vi "TAT_Com_PLC.vi"() -> ()   [LabVIEW 2017]
uses:
  <vilib>/NI/Modbus Library/API/Wrapper/Create TCP Master.vi
  <vilib>/NI/Modbus Library/API/Master/Modbus Master.lvclass
  <vilib>/NI/Modbus Library/API/Wrapper/API Main.lvlib
panel:
  out "Array":i32[](array[numeric])
  out "PLC STATUS":bool
  in  "error in":errorcluster
  in  "stop":bool
  # "Ass & Leak"
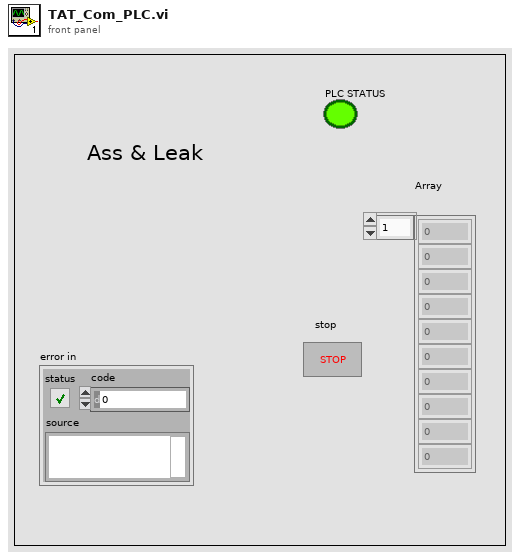
[diagram p1: front panel]
types:
  T1 = enum32{"invalid app kind", "Development System", "Run Time System", "Student Edition", "Embedded LabVIEW", "Evaluation", "Custom"}
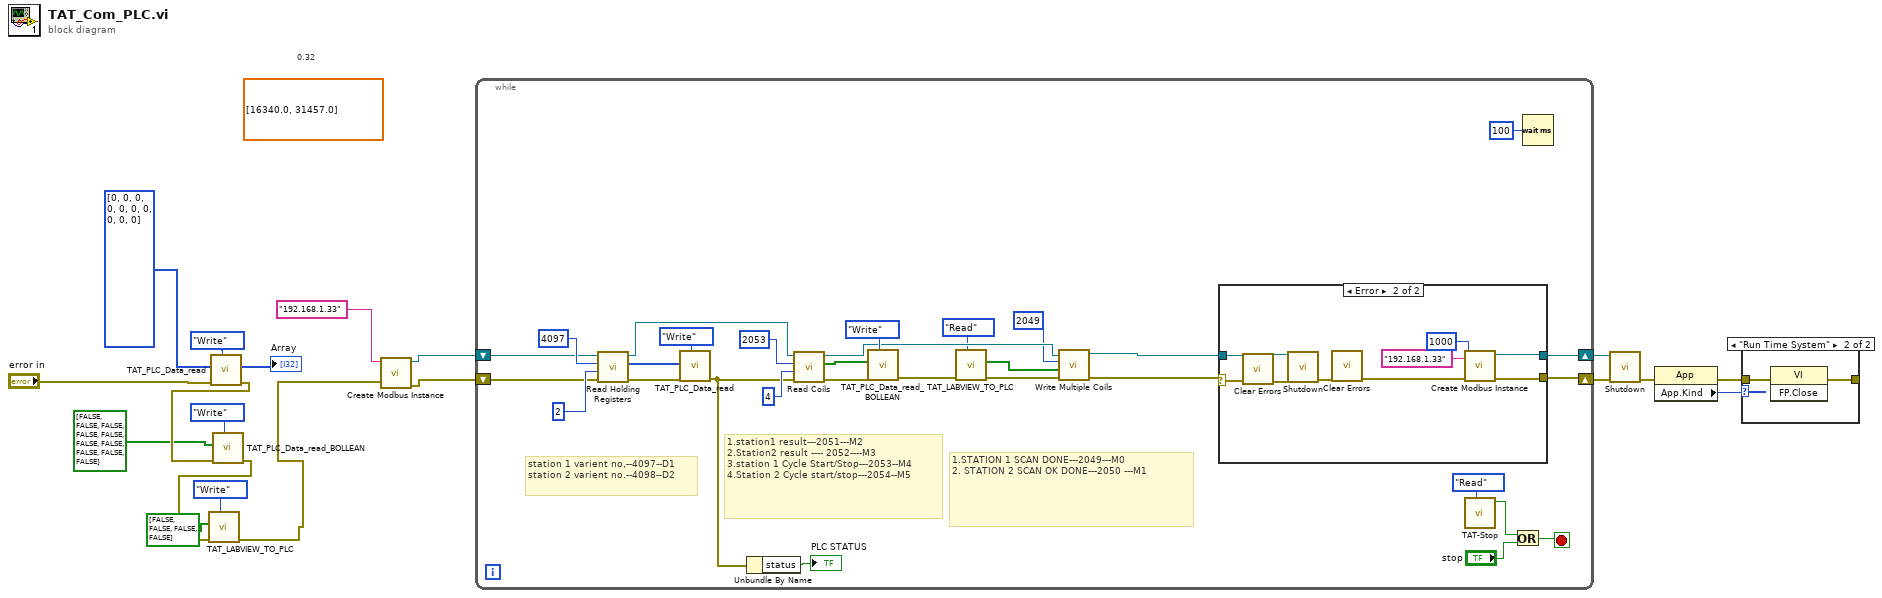
[diagram p0: block diagram]
diagram:
  (unwired) dbl[] [16340.0, 31457.0] ("register values")
  # "0.32"
  n1 = call "TAT_PLC_Data_read.vi"("Enum"=enum16{"Read", "Write"}."Write", "error in (no error)"="error in", "Array"=i64[] [0, 0, 0, 0, 0, 0, 0, 0, 0, 0] ("Array 3")) -> ("error out"=w6:errorcluster, "Array 2"=→"Array":u16[])  [unwired: 7 in]
  n2 = call "TAT_PLC_Data_read_BOLLEAN.vi"("Enum"=enum16{"Read", "Write"}."Write", "error in (no error)"=w6, "Array"=bool[] [FALSE, FALSE, FALSE, FALSE, FALSE, FALSE, FALSE, FALSE, FALSE, FALSE]) -> ("error out"=w2:errorcluster)  [unwired: 7 in, 1 out]
  n3 = call "TAT_LABVIEW_TO_PLC.vi"("Enum"=enum16{"Read", "Write"}."Write", "error in (no error)"=w2, "Array"=bool[] [FALSE, FALSE, FALSE, FALSE]) -> ("error out"=w3:errorcluster)  [unwired: 7 in, 1 out]
  n4 = call-poly <vilib>:"Create Modbus Instance.vi"("error in"=w3, "address"="192.168.1.33") -> ("error out"=w13:errorcluster, "TCP master instance"=w12:refnum<class "Modbus Master.lvclass">)  [unwired: 8 in]
  n5 = while {
    shift-right: [w47] -> w18
    shift-left: w12 -> [w42]
    shift-right: [w46] -> w17
    shift-left: w13 -> [w43]
    stop <- w48 stop-if-true
    # "1.STATION 1 SCAN DONE---2049---M0\n2. STATION 2 SCAN OK DONE---2050 ---M1"
    # "1.station1 result---2051---M2\n2.Station2 result ---- 2052----M3\n3.station 1 Cycle Start/Stop---2053--M4\n4.Station 2 Cycle start/stop---2054--M5"
    # "station 1 varient no,--4097--D1\nstation 2 varient no.--4098--D2"
    n6 = call-dynamic "Read Holding Registers.vi"("error in"=w43, "number of inputs"=u16 2, "starting address"=u16 4097, "Modbus master in"=w42) -> ("error out"=w37:errorcluster, "register values"=w39:u16[], "Modbus master out"=w33:refnum<class "Modbus Master.lvclass">)  [unwired: 5 in]
    n7 = call "TAT_PLC_Data_read.vi"("Enum"=enum16{"Read", "Write"}."Write", "error in (no error)"=w37, "Array"=w39) -> ("error out"=w34:errorcluster)  [unwired: 7 in, 1 out]
    n8 = Unbundle By Name(w34) -> ("status"=→"PLC STATUS":bool)
    n9 = call-dynamic "Read Coils.vi"("error in"=w34, "number of inputs"=u16 4, "starting address"=u16 2053, "Modbus master in"=w33) -> ("error out"=w30:errorcluster, "coils"=w32:bool[], "Modbus master out"=w28:refnum<class "Modbus Master.lvclass">)  [unwired: 5 in]
    n10 = call "TAT_PLC_Data_read_BOLLEAN.vi"("Enum"=enum16{"Read", "Write"}."Write", "error in (no error)"=w30, "Array"=w32) -> ("error out"=w24:errorcluster)  [unwired: 7 in, 1 out]
    n11 = call "TAT_LABVIEW_TO_PLC.vi"("Enum"=enum16{"Read", "Write"}."Read", "error in (no error)"=w24) -> ("error out"=w23:errorcluster, "Array 2"=w25:bool[])  [unwired: 8 in]
    n12 = call-dynamic "Write Multiple Coils.vi"("error in"=w23, "coils to write"=w25, "starting address"=u16 2049, "Modbus master in"=w28) -> ("error out"=w29:errorcluster, "Modbus master out"=w27:refnum<class "Modbus Master.lvclass">)  [unwired: 6 in]
    n13 = case shown="Error" w29 {
      selector: w29 -> [w50 w60]
      tunnel: w27 -> [w51 w58]
      tunnel: [w51 w54] -> w47
      tunnel: [w50 w53] -> w46
      frame No Error {
      }
      frame Error {
        n14 = call <vilib>:"Clear Errors.vi"("error in (no error)"=w60) -> ("error out"=w59:errorcluster)  [unwired: 5 in, 1 out]
        n15 = call-dynamic "Shutdown.vi"("error in"=w59, "Modbus master in"=w58) -> ("error out"=w57:errorcluster)  [unwired: 9 in]
        n16 = call <vilib>:"Clear Errors.vi"("error in (no error)"=w57) -> ("error out"=w55:errorcluster)  [unwired: 5 in, 1 out]
        n17 = call-poly <vilib>:"Create Modbus Instance.vi"("error in"=w55, "connect timeout ms"=1000, "address"="192.168.1.33") -> ("error out"=w53:errorcluster, "TCP master instance"=w54:refnum<class "Modbus Master.lvclass">)  [unwired: 7 in]
      }
    }
    n18 = call "TAT-Stop.vi"("Enum"=enum16{"Read", "Write"}."Read") -> ("Stop"=w20:bool)  [unwired: 10 in]
    n19 = Or(x=w20, y="stop") -> (x .or. y?=w48:bool)
    n20 = Wait (ms)(milliseconds to wait=u32 100) -> ()  [unwired: 1 out]
  }
  n21 = call-dynamic "Shutdown.vi"("error in"=w17, "Modbus master in"=w18) -> ("error out"=w14:errorcluster)  [unwired: 9 in]
  n22 = property class="App"(error in=w14) -> (error out=w15:errorcluster, "App.Kind"=w16:T1)  [unwired: 1 in, 1 out]
  n23 = case shown="\"Run Time System\"" w16 {
    tunnel: w15 -> [w61 w63]
    tunnel: [w61 w62] -> _
    frame Default {
    }
    frame "Run Time System" {
      n24 = invoke class="VI" method="FP.Close"(error in=w63) -> (error out=w62:errorcluster)  [unwired: 2 in, 2 out]
    }
  }
